vi "Flip Flop.vi"(1 "Reset":bool, 2 "Value to be latched":bool) -> (0 "Indicator":bool)   [LabVIEW 2015]
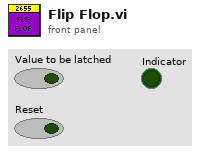
[diagram p1: front panel]
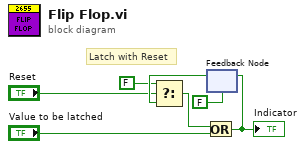
[diagram p0: block diagram]
diagram:
  # "Latch with Reset"
  n1 = feedback #1(FALSE) -> (w3:bool)
  n2 = Select(t=FALSE, s="Reset", f=w3) -> (s? t:f=w4:bool)
  n3 = Or(x=w4, y="Value to be latched") -> (x .or. y?=w7:bool)
  "Indicator" <- w7
  n4 = feedback-in #1(w7) -> ()
